vi "Create Path with Incrementing Suffix.vi"(8 "error in (no error)":errorcluster, 11 "Base Path (in)":path) -> (0 "error out":errorcluster, 2 "Incremented Path":path, 3 "Base Path (out)":path)   [LabVIEW 2016]
uses:
  <userlib>/_OpenG.lib/file/file.llb/Strip Path Extension - String__ogtk.vi
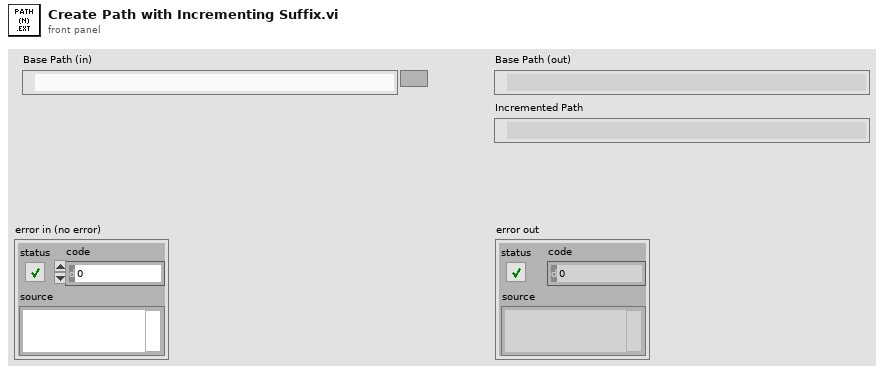
[diagram p1: front panel]
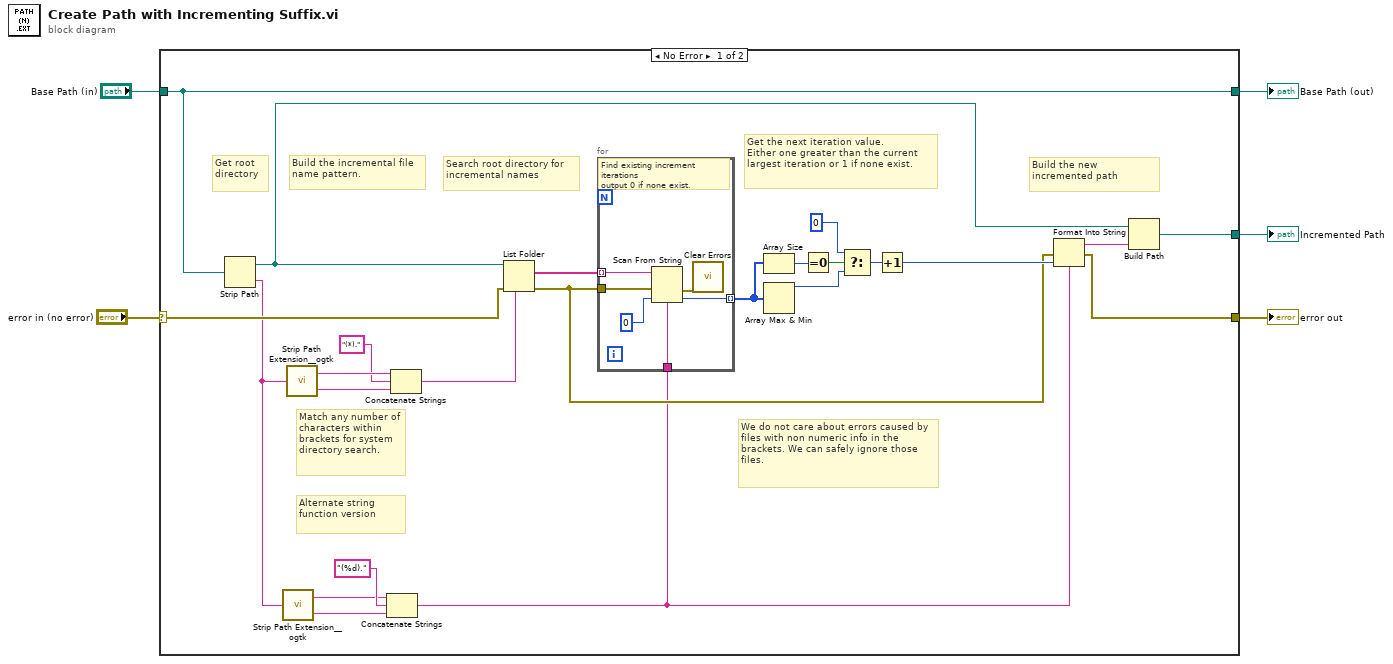
[diagram p0: block diagram]
diagram:
  n1 = case shown="No Error" "error in (no error)" {
    selector: "error in (no error)" -> [w28 w36]
    tunnel: "Base Path (in)" -> [w29 w37]
    tunnel: [w29 w37] -> w3
    tunnel: [w10 w36] -> w2
    tunnel: [w7 _] -> w1
    frame No Error {
      # "We do not care about errors caused by files with non numeric info in the brackets. We can safely ignore those files."
      # "Build the new incremented path"
      # "Get the next iteration value.\nEither one greater than the current largest iteration or 1 if none exist."
      # "Alternate string function version"
      # "Match any number of characters within brackets for system directory search."
      # "Build the incremental file name pattern."
      # "Search root directory for incremental names"
      # "Get root directory"
      n2 = Strip Path(path=w29) -> (stripped path=w8:path, name=w20:string)
      n3 = call-poly <userlib>:"Strip Path Extension__ogtk.vi"("path"=w20) -> ("root"=w22:string, "extension"=w21:string)
      n4 = call-poly <userlib>:"Strip Path Extension__ogtk.vi"("path"=w20) -> ("root"=w27:string, "extension"=w6:string)
      n5 = Concatenate Strings(w22, "(%d).", w21) -> (w11:string)
      n6 = Concatenate Strings(w27, "(*).", w6) -> (w25:string)
      n7 = List Folder(path=w8, pattern=w25, error in=w28) -> (filenames=w24:string[], error out=w12:errorcluster)  [unwired: 1 in, 2 out]
      n8 = for {
        tunnel: w24 -> [w35] mode=indexing
        tunnel: w11 -> [w34]
        tunnel: w12 -> [w32]
        tunnel: [w31] -> w16 mode=indexing
        # "Find existing increment iterations\noutput 0 if none exist."
        n9 = Scan From String(format string=w34, input string=w35, error in=w32, default 1=0) -> (error out=w30:errorcluster, output 1=w31:i32)  [unwired: 1 in, 2 out]
        n10 = call <vilib>:"Clear Errors.vi"("error in (no error)"=w30) -> ()  [unwired: 5 in, 2 out]
      }
      n11 = Array Size(array=w16) -> (size(s)=w19:i32)
      n12 = Array Max & Min(array=w16) -> (max value=w15:i32)  [unwired: 3 out]
      n13 = Equal To 0?(x=w19) -> (x = 0?=w18:bool)
      n14 = Select(t=0, s=w18, f=w15) -> (s? t:f=w14:i32)
      n15 = Increment(x=w14) -> (x+1=w13:i32)
      n16 = Format Into String(format string=w11, error in=w12, w13) -> (resulting string=w9:string, error out=w10:errorcluster)  [unwired: 1 in]
      n17 = Build Path(base path=w8, name or relative path=w9) -> (appended path=w7:path)
    }
    frame Error {
    }
  }
  "Base Path (out)" <- w3
  "Incremented Path" <- w1
  "error out" <- w2
